vi "Aero_tunnel_monitor.vi"() -> ()   [LabVIEW 2010]
panel:
  out "Required WindSpeedRatio":dbl
  out "ROAD SPEED_mps":dbl
  in  "BL Fan1":i32
  in  "BL Fan2":i32
  in  "Stop drive":bool
  in  "Start Drive":bool
  in  "Synch to Wind":bool
  out "Road Info":string
  in  "stop":bool
  out "Lift":dbl caption="N" format="%#.2f"
  out "Pitch":dbl caption="N.m" format="%#.2f"
  out "Drag":dbl caption="N" format="%#.2f"
  out "Side-Force":dbl caption="N" format="%#.2f"
  out "Yaw":dbl caption="N.m" format="%#.2f"
  out "Roll":dbl caption="N.m" format="%#.2f"
  out "SmAD Data":dbl[](array[numeric]) format="%.2f"
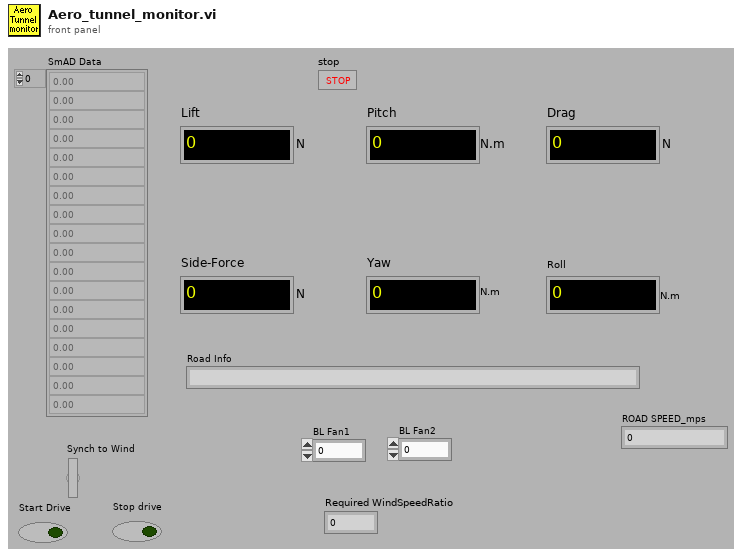
[diagram p1: front panel]
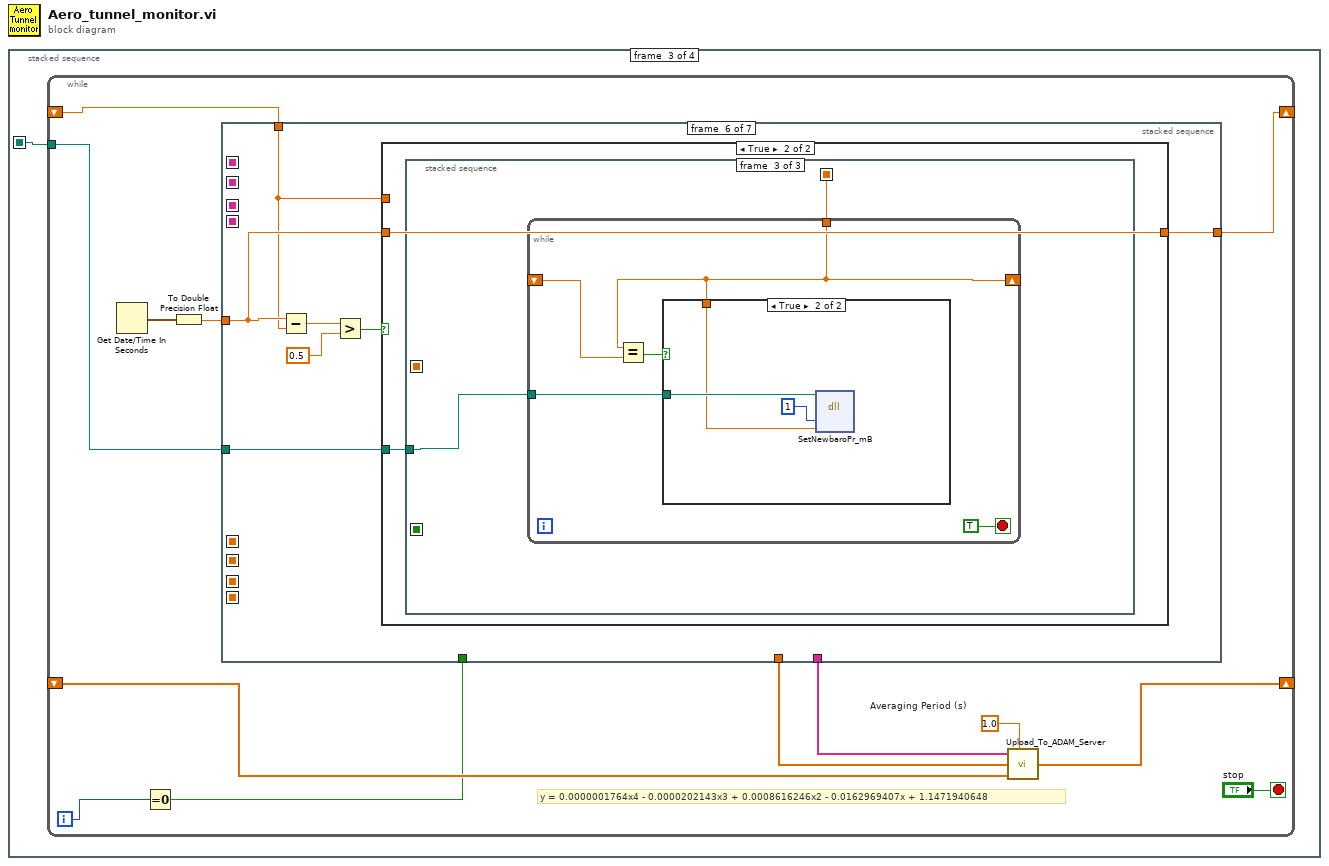
[diagram p0: block diagram]
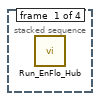
[diagram p2: hidden frame]
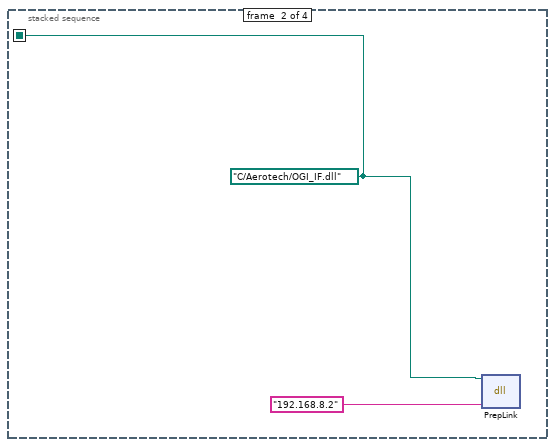
[diagram p3: hidden frame]
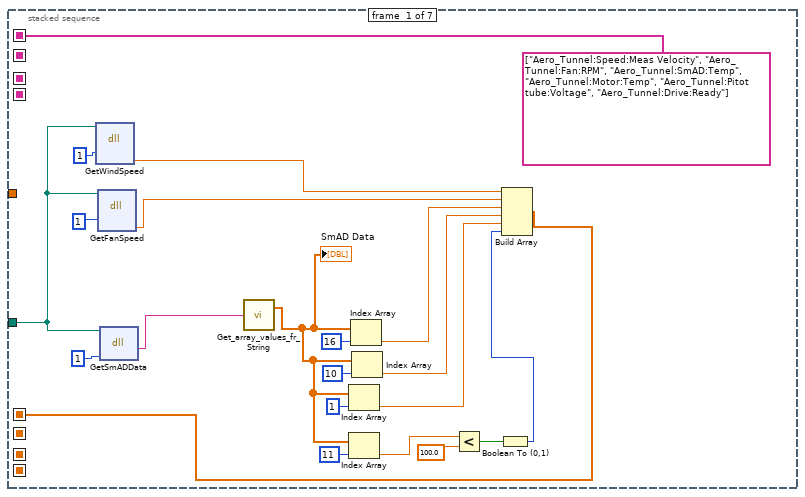
[diagram p4: hidden frame]
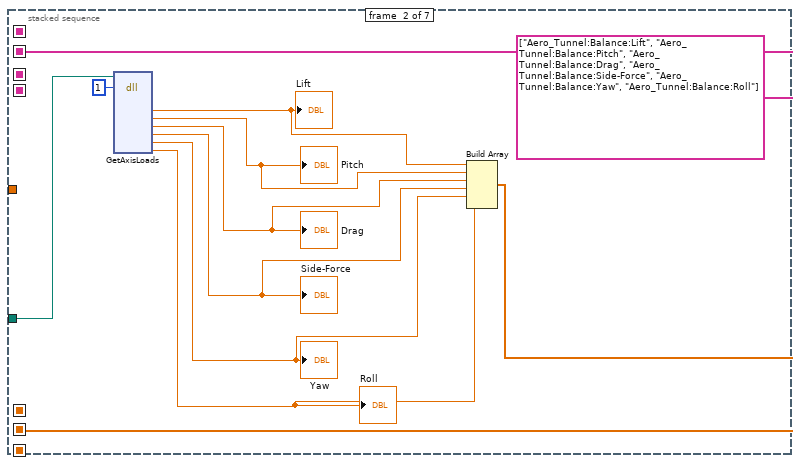
[diagram p5: hidden frame]
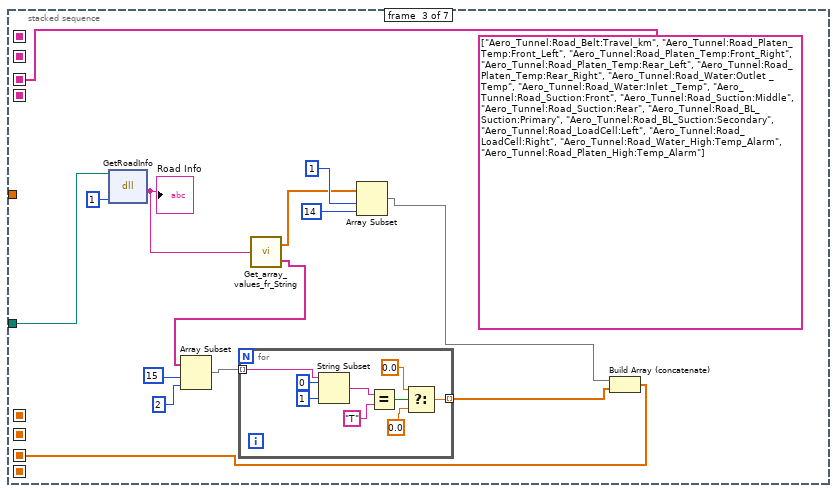
[diagram p6: hidden frame]
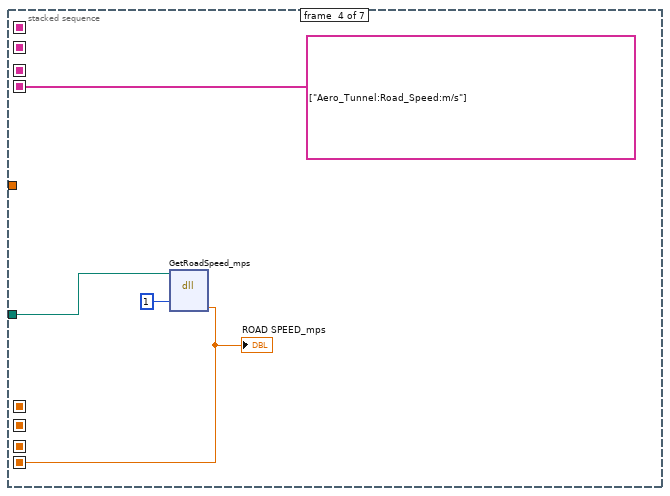
[diagram p7: hidden frame]
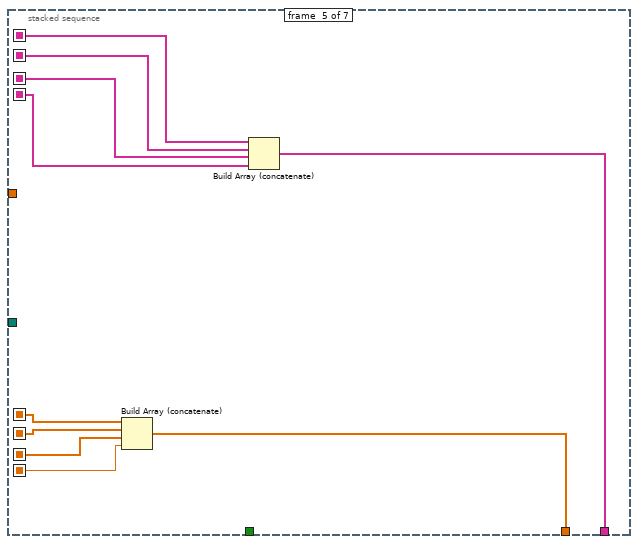
[diagram p8: hidden frame]
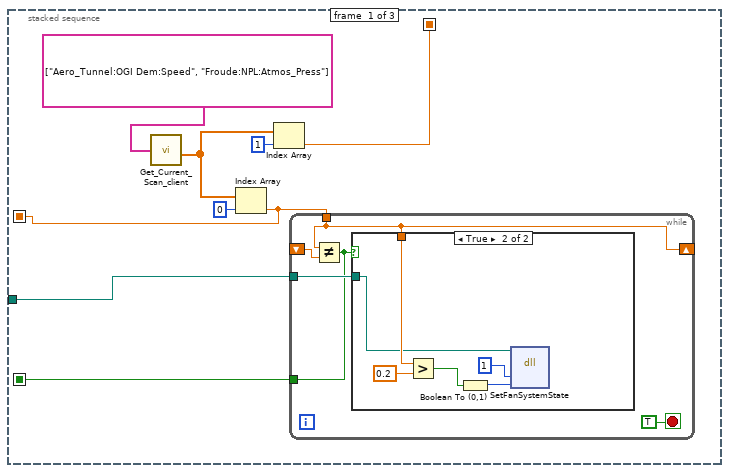
[diagram p10: hidden frame]
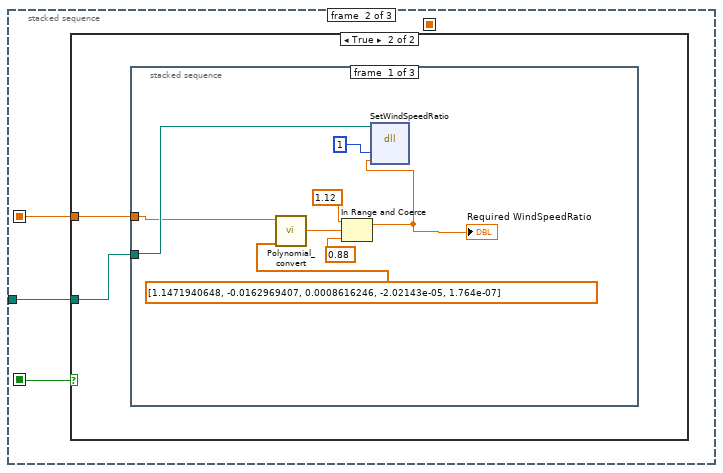
[diagram p12: hidden frame]
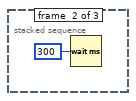
[diagram p14: hidden frame]
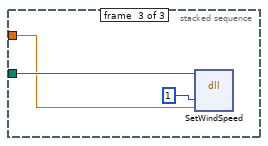
[diagram p15: hidden frame]
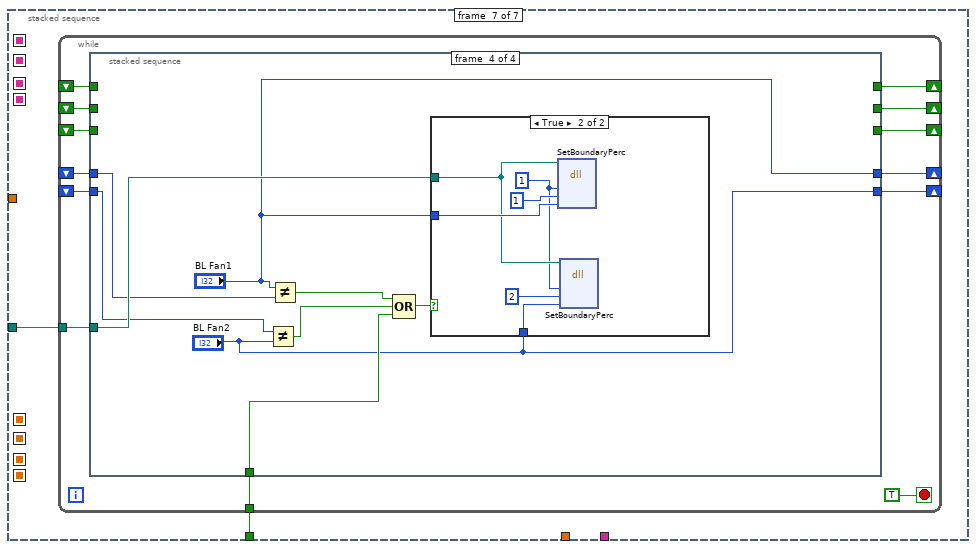
[diagram p17: hidden frame]
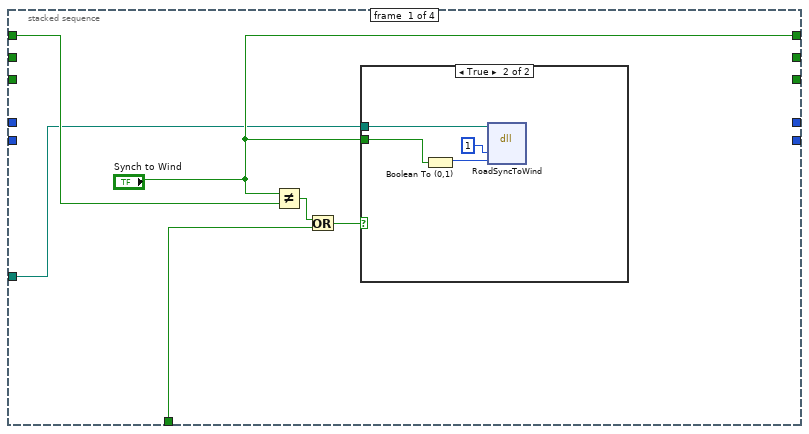
[diagram p18: hidden frame]
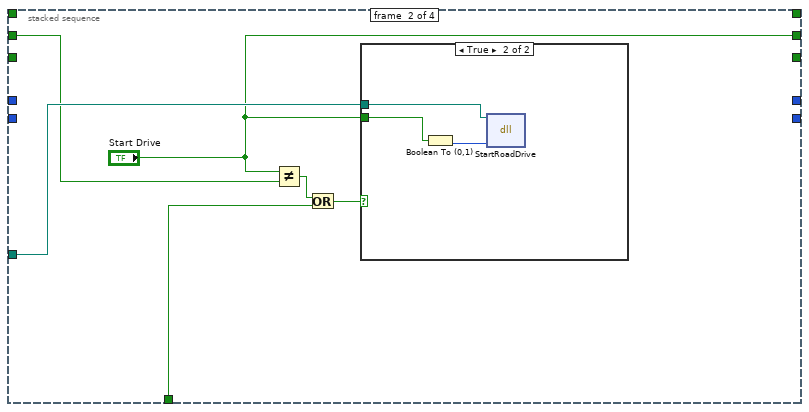
[diagram p20: hidden frame]
diagram:
  n1 = stacked-sequence {
    seq-local: [_ w1 _ _] -> [_ _ w3 w199]
    frame #0 {
      n2 = call "Run_EnFlo_Hub.vi"() -> ()  [unwired: 8 in]
    }
    frame #1 {
      w1 = path "C:/Aerotech/OGI_IF.dll" ("path in")
      n3 = dll-call lib="C:/Aerotech/Drivers/OGI_IF.dll" fn="PrepLink"(path in=w1, "IPAddress"="192.168.8.2") -> ()  [unwired: 2 in, 4 out]
    }
    frame #2 {
      n4 = while {
        shift-right: [w16] -> _
        shift-left: _ -> [w14]
        tunnel: w3 -> [w11]
        shift-right: [w6] -> _
        shift-left: _ -> [w9]
        i -> [w5]
        stop <- "stop" stop-if-true
        w12 = 1.0  # Averaging Period (s)
        # "y = 0.0000001764x4 - 0.0000202143x3 + 0.0008616246x2 - 0.0162969407x + 1.1471940648"
        n5 = Get Date/Time In Seconds() -> (seconds since 1Jan1904=w8:timestamp)
        n6 = Equal To 0?(x=w5) -> (x = 0?=w4:bool)
        n7 = To Double Precision Float(number=w8) -> (double precision float=w7:dbl)
        n8 = stacked-sequence {
          seq-local: [string[] ["Aero_Tunnel:Speed:Meas Velocity", "Aero_Tunnel:Fan:RPM", "Aero_Tunnel:SmAD:Temp", "Aero_Tunnel:Motor:Temp", "Aero_Tunnel:Pitot tube:Voltage", "Aero_Tunnel:Drive:Ready"] ("Channel Names") _ _ _ _ _ _] -> [_ _ _ _ w84 _ _]
          seq-local: [w25 _ _ _ _ _ _] -> [_ _ _ _ w82 _ _]
          seq-local: [_ string[] ["Aero_Tunnel:Balance:Lift", "Aero_Tunnel:Balance:Pitch", "Aero_Tunnel:Balance:Drag", "Aero_Tunnel:Balance:Side-Force", "Aero_Tunnel:Balance:Yaw", "Aero_Tunnel:Balance:Roll"] ("Channel Names") _ _ _ _ _] -> [_ _ _ _ w83 _ _]
          seq-local: [_ w46 _ _ _ _ _] -> [_ _ _ _ w81 _ _]
          seq-local: [_ _ w49 _ _ _ _] -> [_ _ _ _ w77 _ _]
          seq-local: [_ _ string[] ["Aero_Tunnel:Road_Belt:Travel_km", "Aero_Tunnel:Road_Platen_Temp:Front_Left", "Aero_Tunnel:Road_Platen_Temp:Front_Right", "Aero_Tunnel:Road_Platen_Temp:Rear_Left", "Aero_Tunnel:Road_Platen_Temp:Rear_Right", "Aero_Tunnel:Road_Water:Outlet _Temp", "Aero_Tunnel:Road_Water:Inlet _Temp", "Aero_Tunnel:Road_Suction:Front", "Aero_Tunnel:Road_Suction:Middle", "Aero_Tunnel:Road_Suction:Rear", "Aero_Tunnel:Road_BL_Suction:Primary", "Aero_Tunnel:Road_BL_Suction:Secondary", "Aero_Tunnel:Road_LoadCell:Left", "Aero_Tunnel:Road_LoadCell:Right", "Aero_Tunnel:Road_Water_High:Temp_Alarm", "Aero_Tunnel:Road_Platen_High:Temp_Alarm"] ("Channel Names") _ _ _ _] -> [_ _ _ _ w78 _ _]
          seq-local: [_ _ _ string[] ["Aero_Tunnel:Road_Speed:m/s"] ("Channel Names") _ _ _] -> [_ _ _ _ w76 _ _]
          seq-local: [_ _ _ w71 _ _ _] -> [_ _ _ _ w75 _ _]
          tunnel: [_ _ _ _ w80 _ _] -> w15
          tunnel: [_ _ _ _ w79 _ _] -> w13
          tunnel: w11 -> [w17 w44 w60 w73 _ w88 w141]
          tunnel: w7 -> [_ _ _ _ _ w86 _]
          tunnel: w9 -> [_ _ _ _ _ w85 _]
          tunnel: [_ _ _ _ _ w87 _] -> w6
          tunnel: w4 -> [_ _ _ _ _ _ w142]
          frame #0 {
            n9 = dll-call lib="C:/Aerotech/Drivers/OGI_IF.dll" fn="GetWindSpeed"(path in=w17, "Enable"=1) -> ("Windspeed_M/s"=w18:dbl)  [unwired: 3 in, 4 out]
            n10 = dll-call lib="C:/Aerotech/Drivers/OGI_IF.dll" fn="GetFanSpeed"(path in=w17, "Enable"=1) -> ("FanSpeedinRPM"=w19:dbl)  [unwired: 3 in, 4 out]
            n11 = dll-call lib="C:/Aerotech/Drivers/OGI_IF.dll" fn="GetSmADData"(path in=w17, "Enable"=1) -> ("SmAD Data String"=w22:string)  [unwired: 2 in, 3 out]
            n12 = call "Get_array_values_fr_String.vi"("String Value"=w22) -> ("Numeric Array"=w30:dbl[])  [unwired: 1 out]
            "SmAD Data" <- w30
            n13 = Index Array(array=w30, index=1) -> (element=w32:dbl)
            n14 = Index Array(array=w30, index=11) -> (element=w29:dbl)
            n15 = Index Array(array=w30, index=16) -> (element=w35:dbl)
            n16 = Index Array(array=w30, index=10) -> (element=w34:dbl)
            n17 = Less?(x=w29, y=100.0) -> (x < y?=w27:bool)
            n18 = Boolean To (0,1)(Boolean=w27) -> (0, 1=w26:i16)
            n19 = Build Array(w18, w19, w35, w34, w32, w26) -> (w25:dbl[])
          }
          frame #1 {
            n20 = dll-call lib="C:/Aerotech/Drivers/OGI_IF.dll" fn="GetAxisLoads"(path in=w44, "Enable"=1) -> ("Lift"=w43:dbl, "Pitch"=w42:dbl, "Drag"=w41:dbl, "side"=w40:dbl, "Yaw"=w39:dbl, "Roll"=w38:dbl)  [unwired: 3 in, 9 out]
            "Lift" <- w43
            "Pitch" <- w42
            "Drag" <- w41
            "Side-Force" <- w40
            "Yaw" <- w39
            "Roll" <- w38
            n21 = Build Array(w43, w42, w41, w40, w39, w38) -> (w46:dbl[])
          }
          frame #2 {
            n22 = dll-call lib="C:/Aerotech/Drivers/OGI_IF.dll" fn="GetRoadInfo"(path in=w60, "Enable"=1) -> ("Road Info"=w59:string)  [unwired: 3 in, 2 out]
            "Road Info" <- w59
            n23 = call "Get_array_values_fr_String.vi"("String Value"=w59) -> ("Numeric Array"=w56:dbl[], "String array"=w54:string[])
            n24 = Array Subset(array=w54, index=15, length=2) -> (w52:string[])
            n25 = for {
              tunnel: w52 -> [w68] mode=indexing
              tunnel: [w62] -> w51 mode=indexing
              n26 = String Subset(string=w68, offset (0)=0, length (rest)=1 ("length (rest)")) -> (substring=w67:string)
              n27 = Equal?(x=w67, y="T") -> (x = y?=w65:bool)
              n28 = Select(t=0.0, s=w65, f=0.0) -> (s? t:f=w62:dbl)
            }
            n29 = Array Subset(array=w56, index=1, length=14) -> (w50:dbl[])
            n30 = Build Array (concatenate)(w50, w51) -> (w49:dbl[])
          }
          frame #3 {
            n31 = dll-call lib="C:/Aerotech/Drivers/OGI_IF.dll" fn="GetRoadSpeed_mps"(path in=w73, "Enable"=1) -> ("RoadSpeed_mps"=w71:dbl)  [unwired: 3 in, 4 out]
            "ROAD SPEED_mps" <- w71
          }
          frame #4 {
            n32 = Build Array (concatenate)(w82, w81, w77, w75) -> (w80:dbl[])
            n33 = Build Array (concatenate)(w84, w83, w78, w76) -> (w79:string[])
          }
          frame #5 {
            n34 = Subtract(x=w86, y=w85) -> (x-y=w91:dbl)
            n35 = Greater?(x=w91, y=0.5) -> (0:w89:bool)
            n36 = case shown="True" w89 {
              tunnel: w88 -> [_ w94]
              tunnel: [w92 w93] -> w87
              tunnel: w86 -> [_ w93]
              tunnel: w85 -> [w92 _]
              frame False {
              }
              frame True {
                n37 = stacked-sequence {
                  seq-local: [w100 _ _] -> [_ w116 _]
                  seq-local: [w99 _ _] -> [_ w115 _]
                  seq-local: [w95 _ _] -> [_ _ w132]
                  tunnel: w94 -> [w102 w114 w131]
                  frame #0 {
                    n38 = call "Get_Current_Scan_client.vi"("ADAM Ch Names"=string[] ["Aero_Tunnel:OGI Dem:Speed", "Froude:NPL:Atmos_Press"] ("appended array")) -> ("Numerical Values"=w96:dbl[])  [unwired: 1 in, 2 out]
                    n39 = Index Array(array=w96, index=0) -> (element=w100:dbl)
                    n40 = Index Array(array=w96, index=1) -> (element=w95:dbl)
                    n41 = while {
                      tunnel: w102 -> [w107]
                      tunnel: w100 -> [w106]
                      shift-right: [w106] -> _
                      shift-left: _ -> [w105]
                      tunnel: [w103] -> w99
                      stop <- TRUE stop-if-true
                      n42 = Not Equal?(x=w106, y=w105) -> (x != y?=w103:bool)
                      n43 = case shown="True" w103 {
                        tunnel: w107 -> [_ w108]
                        tunnel: w106 -> [_ w109]
                        frame False {
                        }
                        frame True {
                          n44 = Greater?(x=w109, y=0.2) -> (0:w110:bool)
                          n45 = Boolean To (0,1)(Boolean=w110) -> (0, 1=w113:i16)
                          n46 = dll-call lib="C:/Aerotech/Drivers/OGI_IF.dll" fn="SetFanSystemState"(path in=w108, "Enable"=1, "Fan ONOFF"=w113) -> ()  [unwired: 3 in, 4 out]
                        }
                      }
                    }
                  }
                  frame #1 {
                    n47 = case shown="True" w115 {
                      tunnel: w116 -> [_ w117]
                      tunnel: w114 -> [_ w118]
                      frame False {
                      }
                      frame True {
                        n48 = stacked-sequence {
                          tunnel: w118 -> [w124 _ w129]
                          tunnel: w117 -> [w123 _ w128]
                          frame #0 {
                            n49 = call "Polynomial_convert.vi"("Calib constants"=dbl[] [1.1471940648, -0.0162969407, 0.0008616246, -2.02143e-05, 1.764e-07], "Voltage"=w123) -> ("Eng Values"=w122:dbl)  [unwired: 4 in]
                            n50 = In Range and Coerce(upper limit=1.12, x=w122, lower limit=0.88) -> (coerced(x)=w119:dbl)  [unwired: 1 out]
                            "Required WindSpeedRatio" <- w119
                            n51 = dll-call lib="C:/Aerotech/Drivers/OGI_IF.dll" fn="SetWindSpeedRatio"(path in=w124, "Enable"=1 ("t"), "Required WindSpeedRatio"=w119) -> ()  [unwired: 4 in, 3 out]
                          }
                          frame #1 {
                            n52 = Wait (ms)(milliseconds to wait=u32 300) -> ()  [unwired: 1 out]
                          }
                          frame #2 {
                            n53 = dll-call lib="C:/Aerotech/Drivers/OGI_IF.dll" fn="SetWindSpeed"(path in=w129, "Enable"=1 ("t"), "NewWindSpeed"=w128) -> ()  [unwired: 4 in, 3 out]
                          }
                        }
                      }
                    }
                  }
                  frame #2 {
                    n54 = while {
                      shift-right: [w134] -> _
                      shift-left: _ -> [w137]
                      tunnel: w132 -> [w134]
                      tunnel: w131 -> [w135]
                      stop <- TRUE stop-if-true
                      n55 = Equal?(x=w134, y=w137) -> (x = y?=w136:bool)
                      n56 = case shown="True" w136 {
                        tunnel: w135 -> [_ w140]
                        tunnel: w134 -> [_ w138]
                        frame False {
                        }
                        frame True {
                          n57 = dll-call lib="C:/Aerotech/Drivers/OGI_IF.dll" fn="SetNewbaroPr_mB"(path in=w140, "Enable"=1, "NewPressure"=w138) -> ()  [unwired: 3 in, 4 out]
                        }
                      }
                    }
                  }
                }
              }
            }
          }
          frame #6 {
            n58 = while {
              shift-right: [w153] -> _
              shift-left: _ -> [w155]
              tunnel: w142 -> [w154]
              tunnel: w141 -> [w151]
              shift-right: [w149] -> _
              shift-left: _ -> [w150]
              shift-right: [w147] -> _
              shift-left: _ -> [w148]
              shift-right: [w144] -> _
              shift-left: _ -> [w146]
              shift-right: [w143] -> _
              shift-left: _ -> [w145]
              stop <- TRUE stop-if-true
              n59 = stacked-sequence {
                tunnel: w155 -> [w161 _ _ _]
                tunnel: w154 -> [w159 w170 w179 w190]
                tunnel: ["Synch to Wind" _ _ _] -> w153
                tunnel: w151 -> [w156 w168 w177 w192]
                tunnel: w150 -> [_ w167 _ _]
                tunnel: [_ "Start Drive" _ _] -> w149
                tunnel: w148 -> [_ _ w176 _]
                tunnel: [_ _ "Stop drive" _] -> w147
                tunnel: w146 -> [_ _ _ w189]
                tunnel: w145 -> [_ _ _ w186]
                tunnel: [_ _ _ "BL Fan1"] -> w144
                tunnel: [_ _ _ "BL Fan2"] -> w143
                frame #0 {
                  n60 = Not Equal?(x="Synch to Wind", y=w161) -> (x != y?=w160:bool)
                  n61 = Or(x=w160, y=w159) -> (x .or. y?=w157:bool)
                  n62 = case shown="True" w157 {
                    tunnel: "Synch to Wind" -> [_ w163]
                    tunnel: w156 -> [_ w162]
                    frame False {
                    }
                    frame True {
                      n63 = Boolean To (0,1)(Boolean=w163) -> (0, 1=w164:i16)
                      n64 = dll-call lib="C:/Aerotech/Drivers/OGI_IF.dll" fn="RoadSyncToWind"(path in=w162, "Enable"=1, "SynchState"=w164) -> ()  [unwired: 3 in, 4 out]
                    }
                  }
                }
                frame #1 {
                  n65 = Not Equal?(x="Start Drive", y=w167) -> (x != y?=w171:bool)
                  n66 = Or(x=w171, y=w170) -> (x .or. y?=w169:bool)
                  n67 = case shown="True" w169 {
                    tunnel: "Start Drive" -> [_ w174]
                    tunnel: w168 -> [_ w172]
                    frame False {
                    }
                    frame True {
                      n68 = Boolean To (0,1)(Boolean=w174) -> (0, 1=w173:i16)
                      n69 = dll-call lib="C:/Aerotech/Drivers/OGI_IF.dll" fn="StartRoadDrive"(path in=w172, "Enable"=w173) -> ()  [unwired: 2 in, 4 out]
                    }
                  }
                }
                frame #2 {
                  n70 = Not Equal?(x="Stop drive", y=w176) -> (x != y?=w180:bool)
                  n71 = Or(x=w180, y=w179) -> (x .or. y?=w178:bool)
                  n72 = case shown="True" w178 {
                    tunnel: "Stop drive" -> [_ w183]
                    tunnel: w177 -> [_ w181]
                    frame False {
                    }
                    frame True {
                      n73 = Boolean To (0,1)(Boolean=w183) -> (0, 1=w182:i16)
                      n74 = dll-call lib="C:/Aerotech/Drivers/OGI_IF.dll" fn="RoadStop"(path in=w181, "Enable"=w182) -> ()  [unwired: 2 in, 4 out]
                    }
                  }
                }
                frame #3 {
                  n75 = Not Equal?(x=w186, y="BL Fan2") -> (x != y?=w187:bool)
                  n76 = Not Equal?(x="BL Fan1", y=w189) -> (x != y?=w188:bool)
                  n77 = Compound Arithmetic op=OR(w188, w187, w190) -> (w191:bool)
                  n78 = case shown="True" w191 {
                    tunnel: w192 -> [_ w194]
                    tunnel: "BL Fan1" -> [_ w196]
                    tunnel: "BL Fan2" -> [_ w195]
                    frame False {
                    }
                    frame True {
                      w193 = 1 ("BL Fan (1 or 2)")
                      n79 = dll-call lib="C:/Aerotech/Drivers/OGI_IF.dll" fn="SetBoundaryPerc"(path in=w194, "enable"=w193, "BL Fan (1 or 2)"=1, "New Percentage"=w196) -> ()  [unwired: 4 in, 4 out]
                      n80 = dll-call lib="C:/Aerotech/Drivers/OGI_IF.dll" fn="SetBoundaryPerc"(path in=w194, "enable"=w193, "BL Fan (1 or 2)"=2, "New Percentage"=w195) -> ()  [unwired: 4 in, 4 out]
                    }
                  }
                }
              }
            }
          }
        }
        n81 = call "Upload_To_ADAM_Server.vi"("Channel Names"=w13, "Averaging Period (s)"=w12, "Channel Values"=w15, "Shift In"=w14) -> ("Shift Out"=w16:dbl[])  [unwired: 1 out]
      }
    }
    frame #3 {
      n82 = dll-call lib="C:/Aerotech/Drivers/OGI_IF.dll" fn="CloseLink"(path in=w199) -> ()  [unwired: 2 in, 3 out]
    }
  }
